vi "Szybka_buforuj.vi"(6 "size(32000)":i32=32000, 7 "#cores (1)":i32=1, 8 "error in (no error)":errorcluster, 9 "Bufor in":T1, 11 "Kanaly in":T1) -> (0 "error out":errorcluster, 1 "Bufor out":T1, 3 "Enk rozm":i32)   [LabVIEW 2013]
doc: "Buforuje próbki w rejestracji szybkiej"
uses:
  Kontrolki/Przetwarzanie/Kanaly.ctl
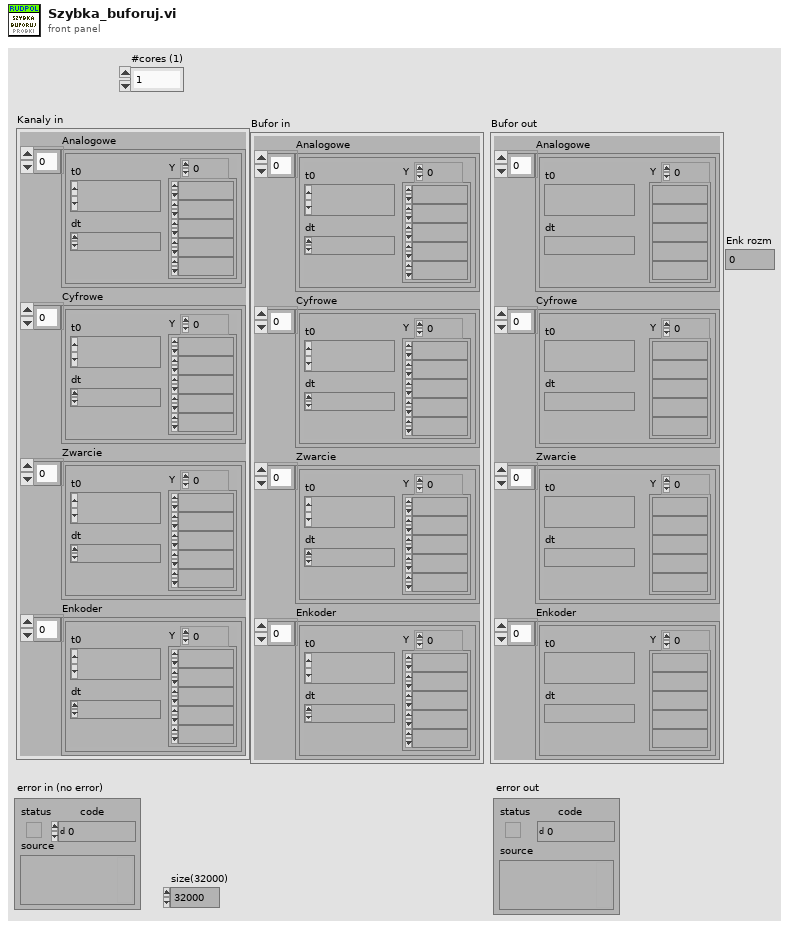
[diagram p1: front panel]
types:
  T1 = typedef "Kanaly.ctl" = cluster{"Analogowe":waveform(dbl)[], "Cyfrowe":waveform(dbl)[], "Zwarcie":waveform(dbl)[], "Enkoder":waveform(dbl)[]}
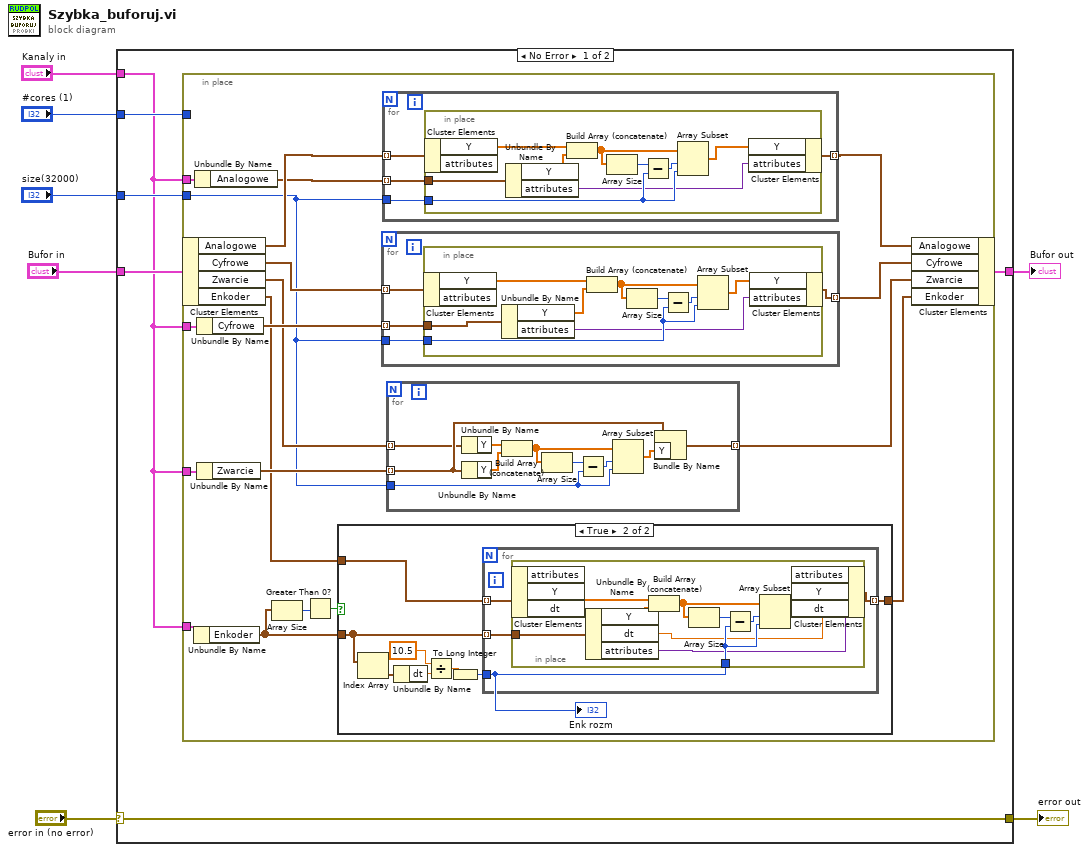
[diagram p0: block diagram]
diagram:
  n1 = case shown="No Error" "error in (no error)" {
    selector: "error in (no error)" -> [w10 w93]
    tunnel: [w10 w93] -> w6
    tunnel: "Bufor in" -> [w9 w92]
    tunnel: "Kanaly in" -> [w8 _]
    tunnel: [w13 w92] -> w3
    tunnel: "size(32000)" -> [w12 _]
    tunnel: "#cores (1)" -> [w11 _]
    frame No Error {
      n2 = in-place {
        in-place-border: w8 -> [w32]
        in-place-border: w12 -> [w18]
        in-place-border: w11 -> [_]
        in-place-border: w8 -> [w31]
        in-place-border: w8 -> [w29]
        in-place-border: w8 -> [w23]
        n3 = in-place-cluster #1(w9) -> ("Analogowe"=w21:waveform(dbl)[], "Cyfrowe"=w27:waveform(dbl)[], "Zwarcie"=w26:waveform(dbl)[], "Enkoder"=w14:waveform(dbl)[])
        n4 = Unbundle By Name(w23) -> ("Enkoder"=w17:waveform(dbl)[])
        n5 = Unbundle By Name(w32) -> ("Analogowe"=w20:waveform(dbl)[])
        n6 = Unbundle By Name(w31) -> ("Cyfrowe"=w30:waveform(dbl)[])
        n7 = Unbundle By Name(w29) -> ("Zwarcie"=w28:waveform(dbl)[])
        n8 = Array Size(array=w17) -> (size(s)=w16:i32)
        n9 = Greater Than 0?(x=w16) -> (x > 0?=w15:bool)
        n10 = case shown="True" w15 {
          tunnel: [w33 w41] -> w22
          tunnel: w17 -> [_ w39]
          tunnel: w14 -> [w33 w40]
          frame False {
          }
          frame True {
            n11 = Index Array(array=w39) -> (element=w38:waveform(dbl))  [unwired: 1 in]
            n12 = Unbundle By Name(w38) -> ("dt"=w37:dbl)
            n13 = Divide(x=10.5 ("size(32000)"), y=w37) -> (x/y=w35:dbl)
            n14 = To Long Integer(number=w35) -> (32bit integer=w34:i32)
            "Enk rozm" <- w34
            n15 = for {
              tunnel: w39 -> [w45] mode=indexing
              tunnel: [w42] -> w41 mode=indexing
              tunnel: w40 -> [w43] mode=indexing
              tunnel: w34 -> [w44]
              n16 = in-place {
                in-place-border: w45 -> [w54]
                in-place-border: w44 -> [w50]
                n17 = in-place-cluster #2(w43) -> ("Y"=w48:dbl[])  [unwired: 2 out]
                n18 = Unbundle By Name(w54) -> ("Y"=w55:dbl[], "dt"=w47:dbl, "attributes"=w46:variant)
                n19 = Build Array (concatenate)(w48, w55) -> (w53:dbl[])
                n20 = Array Size(array=w53) -> (size(s)=w52:i32)
                n21 = Subtract(x=w52, y=w50) -> (x-y=w51:i32)
                n22 = Array Subset(array=w53, index=w51, length=w50) -> (w49:dbl[])
                n23 = in-place-cluster #2("attributes"=w46, "Y"=w49, "dt"=w47) -> (w42:waveform(dbl))
              }
            }
          }
        }
        n24 = for {
          tunnel: w30 -> [w82] mode=indexing
          tunnel: [w79] -> w25 mode=indexing
          tunnel: w18 -> [w81]
          tunnel: w27 -> [w80] mode=indexing
          n25 = in-place {
            in-place-border: w82 -> [w90]
            in-place-border: w81 -> [w86]
            n26 = in-place-cluster #3(w80) -> ("Y"=w84:dbl[])  [unwired: 1 out]
            n27 = Unbundle By Name(w90) -> ("Y"=w91:dbl[], "attributes"=w83:variant)
            n28 = Build Array (concatenate)(w84, w91) -> (w89:dbl[])
            n29 = Array Size(array=w89) -> (size(s)=w88:i32)
            n30 = Subtract(x=w88, y=w86) -> (x-y=w87:i32)
            n31 = Array Subset(array=w89, index=w87, length=w86) -> (w85:dbl[])
            n32 = in-place-cluster #3("Y"=w85, "attributes"=w83) -> (w79:waveform(dbl))
          }
        }
        n33 = for {
          tunnel: w20 -> [w59] mode=indexing
          tunnel: [w56] -> w19 mode=indexing
          tunnel: w18 -> [w58]
          tunnel: w21 -> [w57] mode=indexing
          n34 = in-place {
            in-place-border: w59 -> [w67]
            in-place-border: w58 -> [w63]
            n35 = in-place-cluster #4(w57) -> ("Y"=w62:dbl[])  [unwired: 1 out]
            n36 = Unbundle By Name(w67) -> ("Y"=w68:dbl[], "attributes"=w60:variant)
            n37 = Build Array (concatenate)(w62, w68) -> (w66:dbl[])
            n38 = Array Size(array=w66) -> (size(s)=w65:i32)
            n39 = Subtract(x=w65, y=w63) -> (x-y=w64:i32)
            n40 = Array Subset(array=w66, index=w64, length=w63) -> (w61:dbl[])
            n41 = in-place-cluster #4("Y"=w61, "attributes"=w60) -> (w56:waveform(dbl))
          }
        }
        n42 = for {
          tunnel: w28 -> [w77] mode=indexing
          tunnel: [w76] -> w24 mode=indexing
          tunnel: w18 -> [w71]
          tunnel: w26 -> [w70] mode=indexing
          n43 = Unbundle By Name(w70) -> ("Y"=w69:dbl[])
          n44 = Unbundle By Name(w77) -> ("Y"=w78:dbl[])
          n45 = Build Array (concatenate)(w69, w78) -> (w74:dbl[])
          n46 = Array Size(array=w74) -> (size(s)=w73:i32)
          n47 = Subtract(x=w73, y=w71) -> (x-y=w72:i32)
          n48 = Array Subset(array=w74, index=w72, length=w71) -> (w75:dbl[])
          n49 = Bundle By Name(cluster=w77, "Y"=w75) -> (w76:waveform(dbl))
        }
        n50 = in-place-cluster #1("Analogowe"=w19, "Cyfrowe"=w25, "Zwarcie"=w24, "Enkoder"=w22) -> (w13:T1)
      }
    }
    frame Error {
    }
  }
  "error out" <- w6
  "Bufor out" <- w3
